vi "HAPS_LoadTable_SetBeam_Manual_Selected.vi"() -> ()   [LabVIEW 2023, in "HAPS.lvlib"]
uses:
  HAPS.lvlib
  set_ele.ctl
  HAPS_SerialPort.ctl
  HAPS_MCU_ELE_Func.ctl
  <vilib>/Utility/file.llb/Read Delimited Spreadsheet (string).vi
  R_S/R_S.lvlib
panel:
  out "error IO":errorcluster
  out "Err_code":i32
  out "status":bool
  in  "offset?":bool
  in  "simu.?":bool
  in  "set_ele":T1={"ch"=0, "chain_id"=0, "group"=0, "array_id"=0, "ele_phase"=0, "ele_gain"=35, "com_gain"=17, "pd_range"=0}
  in  "ele_gain":i32=35
  in  "BFIC_id?":i32
  in  "Group?":i32
  in  "sys reboot?":bool=TRUE
  in  "VISA resource name":refnum<visa-resource-name>="COM1"
  in  "file path":path=path "D:/_Project/_Code/LabVIEW/_CLC_Gen4/CLC_LV2023/CLC_Cali/Log/HAPS/Preset.csv"
  out "Remaining quantity":i32
  out "ele phase":i32
  out "ele gain":i32
  out "channel":i32
  out "chain ID":i32
  out "group":i32
  out "array id":i32
  # "HAPS 24x24 Setting Manual In-Phase : \n                                                           One BFIC"
  # "Tx:35\nRx:22"
  # "Not using!!!!!!!!!!!!!!!!!!!!!!!!!!!!!!!!!!!!!!!!"
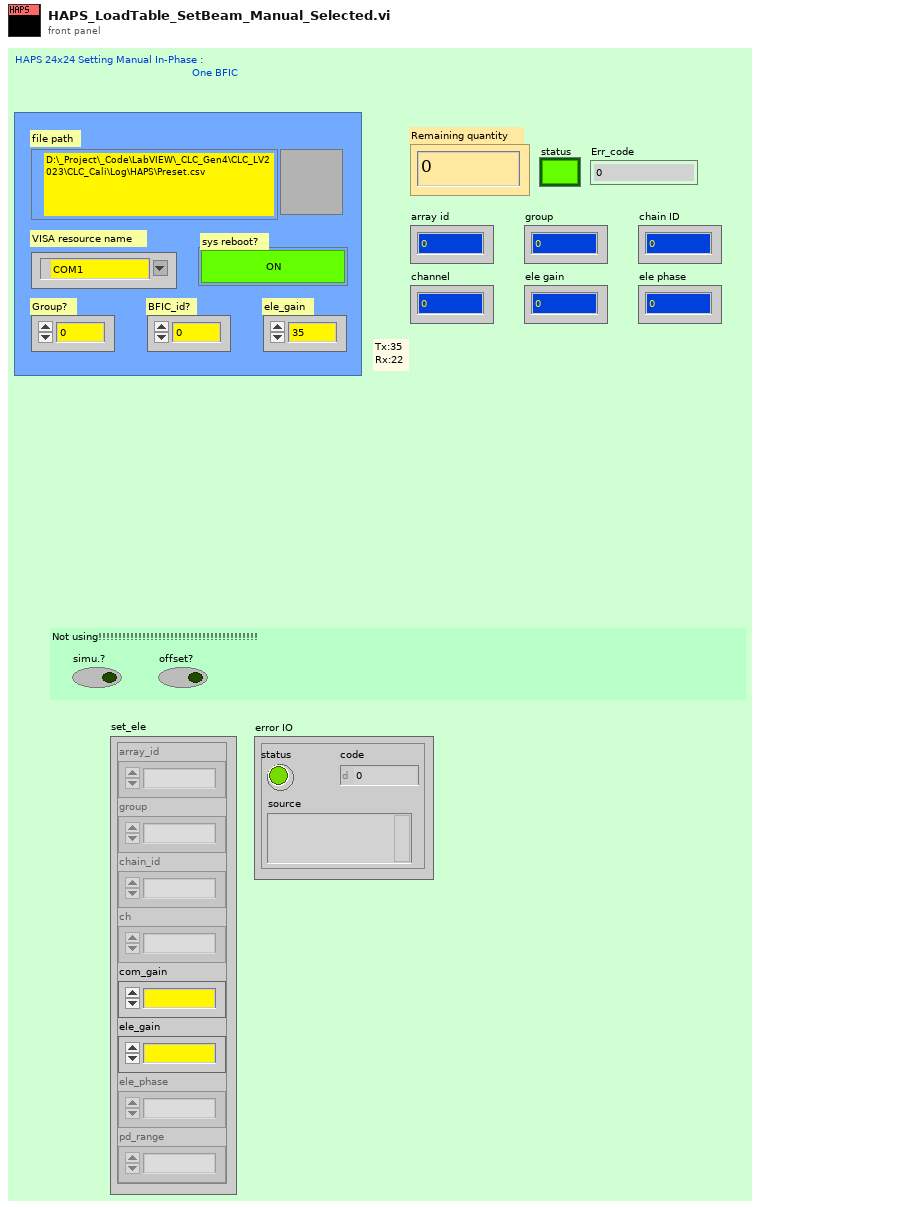
[diagram p1: front panel]
types:
  T1 = typedef "HAPS.lvlib/set_ele.ctl" = cluster{"ch":i32, "chain_id":i32, "group":i32, "array_id":i32, "ele_phase":i32, "ele_gain":i32, "com_gain":i32, "pd_range":i32}
  T2 = typedef "HAPS.lvlib/HAPS_SerialPort.ctl" = enum16{"Init", "Close", "CMD", "Flush"}
  T3 = typedef "HAPS.lvlib/HAPS_MCU_ELE_Func.ctl" = enum16{"array_init", "set_com_gain", "set_ch_gain_phase", "set_pd_range", "get_preamp_temp", "get_bfic_temp", "get_tx_pd", "ch_on", "ch_on_2", "ch_ctrl_all", "array_ctrl_src"}
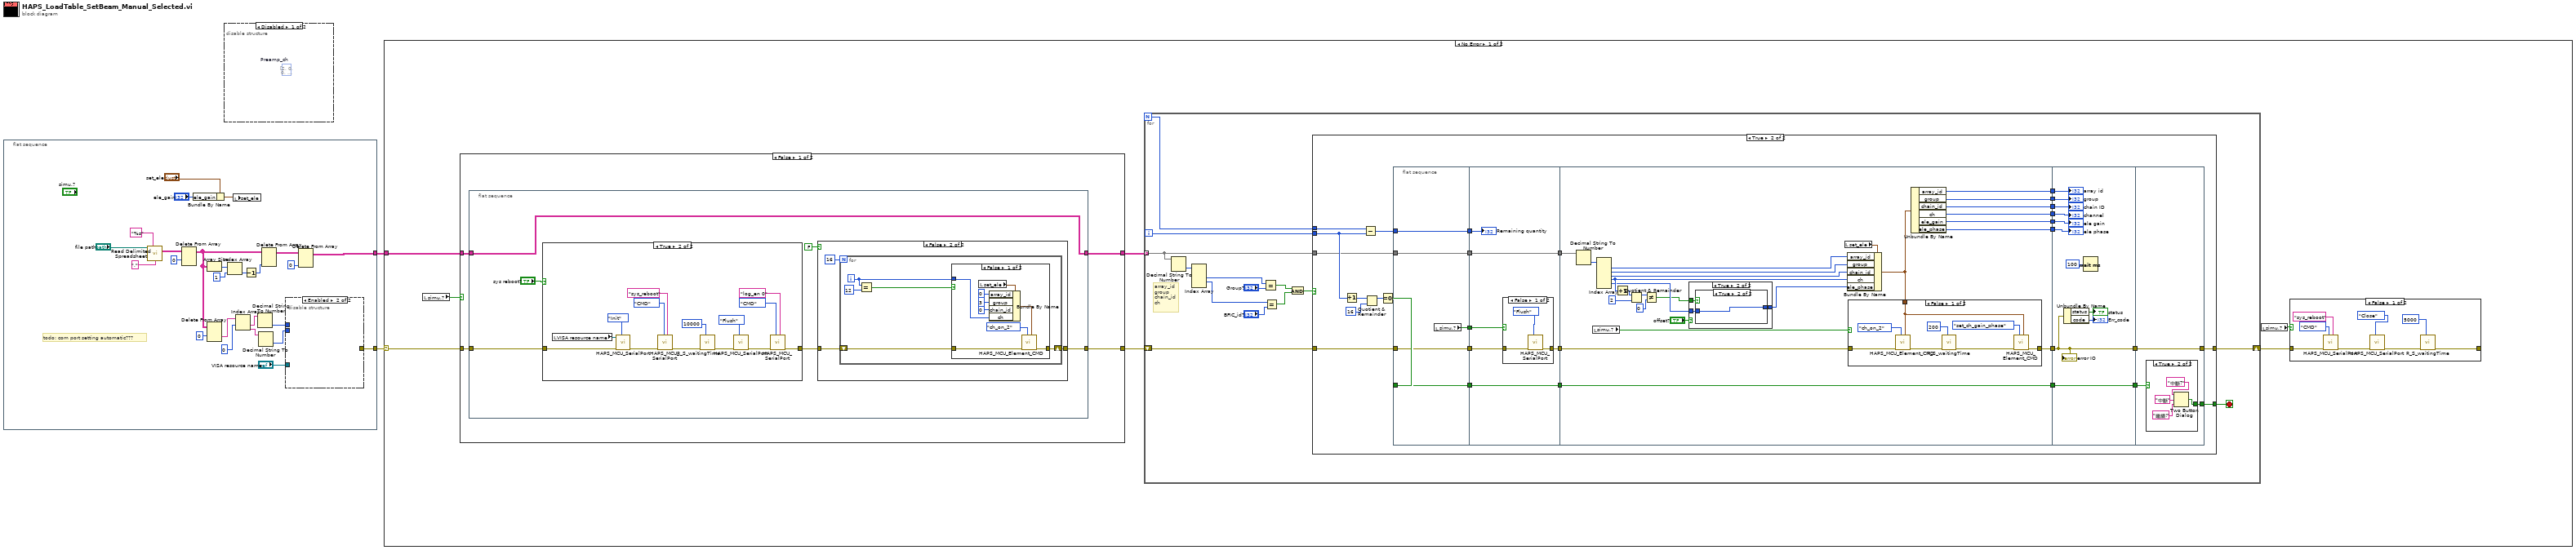
[diagram p0: block diagram]
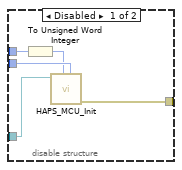
[diagram p2: hidden frame]
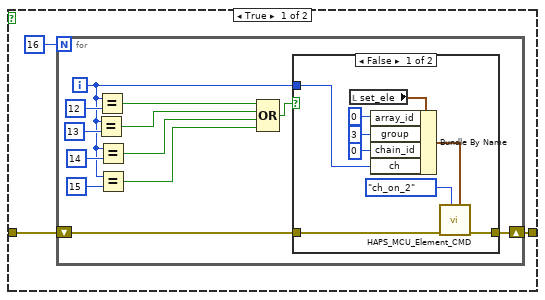
[diagram p5: hidden frame]
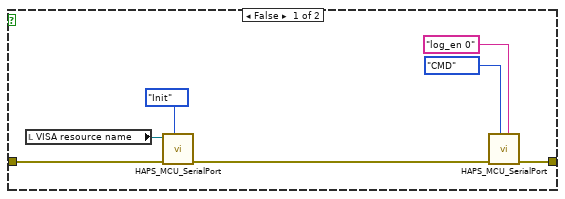
[diagram p8: hidden frame]
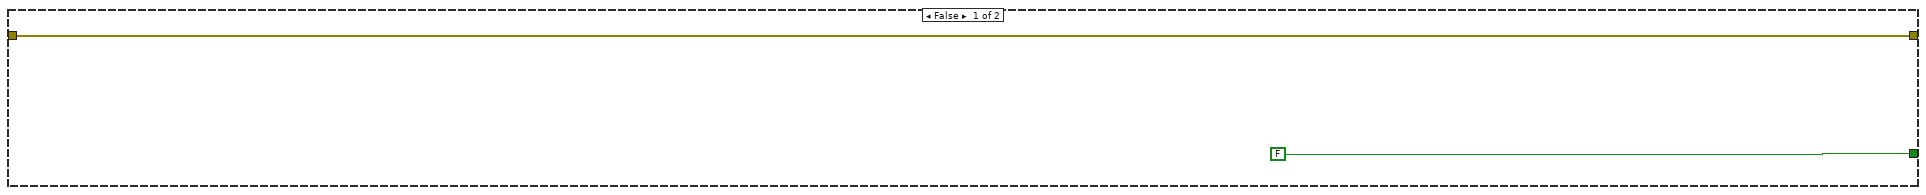
[diagram p10: hidden frame]
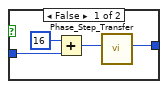
[diagram p13: hidden frame]
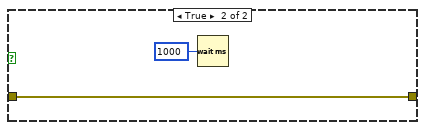
[diagram p14: hidden frame]
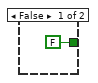
[diagram p15: hidden frame]
diagram:
  n1 = flat-sequence {
    tunnel: [w19] -> w2
    tunnel: [w6] -> w1
    frame #0 {
      # "todo: com port setting automatic???"
      n2 = call-poly <vilib>:"Read Delimited Spreadsheet.vi"("file path (dialog if empty)"="file path", "format (%s)"="%s" ("format (%.3f)"), "delimiter (\\t)"="," ("delimiter (\\t)")) -> ("all rows"=w25:string[][])  [unwired: 7 in, 5 out]
      n3 = Delete From Array(array=w25, index (row)=0) -> (array with subset deleted=w15:string[][])  [unwired: 2 in, 1 out]
      n4 = Bundle By Name(cluster="set_ele", "ele_gain"="ele_gain") -> (w3:T1)
      n5 = Array Size(array=w15) -> (size(s)=w23:i32[])
      n6 = Delete From Array(array=w15, index (row)=0) -> (deleted portion=w14:string[])  [unwired: 2 in, 1 out]
      n7 = Index Array(array=w23, index=1) -> (element=w20:i32)
      n8 = local write "set_ele"(w3) -> ()
      n9 = Index Array(array=w14, index #1=0 ("index")) -> (element #1=w13:string, element #2=w12:string)  [unwired: 1 in]
      n10 = Decrement(x=w20) -> (x-1=w22:i32)
      n11 = Decimal String To Number(string=w13) -> (number=w9:i32)  [unwired: 2 in, 1 out]
      n12 = Decimal String To Number(string=w12) -> (number=w8:i32)  [unwired: 2 in, 1 out]
      n13 = Delete From Array(array=w15, index (col)=w22) -> (array with subset deleted=w18:string[][])  [unwired: 2 in, 1 out]
      n14 = disable-structure shown="Enabled" {
        disable-tunnel: [w32 _] -> w19
        disable-tunnel: w9 -> [w31 _]
        disable-tunnel: w8 -> [w30 _]
        disable-tunnel: "VISA resource name" -> [w29 _]
        frame Disabled {
          n15 = To Unsigned Word Integer(number=w31) -> (unsigned 16bit integer=w28:u16)
          n16 = call "HAPS_MCU_Init.vi"("array_id"=w30, "Tx/Rx"=w28, "VISA resource name"=w29) -> ("error out"=w32:errorcluster)  [unwired: 8 in]
        }
        frame Enabled {
        }
      }
      n17 = Delete From Array(array=w18, index (col)=0 ("index (row)")) -> (array with subset deleted=w6:string[][])  [unwired: 2 in, 1 out]
    }
  }
  n18 = disable-structure shown="Disabled" {
    frame Disabled {
      (unwired) i32[][] [[2, 0, 0, 8, 8, 10, 11, 9, 9, 1, 1, 3], [3, 1, 1, 9, 9, 11, 13, 15, 15, 7, 7, 5], [5, 7, 7, 15, 15, 13, 14, 14, 6, 6, 4, 12]]  # Preamp_ch
    }
    frame Enabled {
    }
  }
  n19 = case shown="No Error" w2 {
    selector: w2 -> [w37 _]
    tunnel: w1 -> [w39 _]
    frame No Error {
      n20 = local read "simu.?"() -> (w35:bool)
      n21 = case shown="False" w35 {
        tunnel: w39 -> [w52 w124]
        tunnel: [w51 w124] -> w38
        tunnel: w37 -> [w50 w123]
        tunnel: [w49 w123] -> w36
        frame False {
          n22 = flat-sequence {
            tunnel: w52 -> [w58]
            tunnel: [w58] -> w51
            tunnel: w50 -> [w56]
            tunnel: [w57] -> w49
            frame #0 {
              n23 = case shown="True" "sys reboot?" {
                tunnel: w56 -> [w106 w120]
                tunnel: [w104 w118] -> w55
                frame False {
                  n24 = local read "VISA resource name"() -> (w102:refnum<visa-resource-name>)
                  n25 = call "HAPS_MCU_SerialPort.vi"("HAPS_SerialPort_Func"=HAPS_SerialPort."Init", "error in"=w106, "VISA resource name"=w102) -> ("error out"=w103:errorcluster)  [unwired: 6 in, 2 out]
                  n26 = call "HAPS_MCU_SerialPort.vi"("Command"="log_en 0", "HAPS_SerialPort_Func"=enum16{"Init", "Close", "CMD"}."CMD" ("HAPS_SerialPort"), "error in"=w103) -> ("error out"=w104:errorcluster)  [unwired: 6 in, 2 out]
                }
                frame True {
                  n27 = local read "VISA resource name"() -> (w109:refnum<visa-resource-name>)
                  n28 = call "HAPS_MCU_SerialPort.vi"("HAPS_SerialPort_Func"=HAPS_SerialPort."Init", "error in"=w120, "VISA resource name"=w109) -> ("error out"=w115:errorcluster)  [unwired: 6 in, 2 out]
                  n29 = call "HAPS_MCU_SerialPort.vi"("Command"="sys_reboot", "HAPS_SerialPort_Func"=enum16{"Init", "Close", "CMD"}."CMD" ("HAPS_SerialPort"), "error in"=w115) -> ("error out"=w114:errorcluster)  [unwired: 6 in, 2 out]
                  n30 = call "R_S_waitingTime.vi"("Waiting Time(ms)"=u32 10000, "error in"=w114) -> ("error out"=w112:errorcluster)  [unwired: 9 in]
                  n31 = call "HAPS_MCU_SerialPort.vi"("HAPS_SerialPort_Func"=HAPS_SerialPort."Flush", "error in"=w112) -> ("error out"=w110:errorcluster)  [unwired: 7 in, 2 out]
                  n32 = call "HAPS_MCU_SerialPort.vi"("Command"="log_en 0", "HAPS_SerialPort_Func"=enum16{"Init", "Close", "CMD"}."CMD" ("HAPS_SerialPort"), "error in"=w110) -> ("error out"=w118:errorcluster)  [unwired: 6 in, 2 out]
                }
              }
              n33 = case shown="False" FALSE {
                tunnel: [w60 w85] -> w57
                tunnel: w55 -> [w59 w84]
                frame True {
                  n34 = for {
                    N: 16 -> [_]
                    shift-right: [w72] -> w60
                    shift-left: w59 -> [w73]
                    i -> [w63]
                    n35 = Equal?(x=w63, y=13) -> (x = y?=w67:bool)
                    n36 = Equal?(x=w63, y=12) -> (x = y?=w71:bool)
                    n37 = Equal?(x=w63, y=14) -> (x = y?=w65:bool)
                    n38 = Equal?(x=w63, y=15) -> (x = y?=w62:bool)
                    n39 = Compound Arithmetic op=OR(w71, w67, w65, w62) -> (w68:bool)
                    n40 = case shown="False" w68 {
                      tunnel: w73 -> [w76 w83]
                      tunnel: [w75 w83] -> w72
                      tunnel: w63 -> [w74 _]
                      frame False {
                        n41 = local read "set_ele"() -> (w78:T1)
                        n42 = Bundle By Name(cluster=w78, "array_id"=0, "group"=3, "chain_id"=0, "ch"=w74) -> (w79:T1)
                        n43 = call "HAPS_MCU_Element_CMD.vi"("set_ele"=w79, "HAPS_MCU_ELE_Func."=HAPS_MCU_ELE_Func."ch_on_2", "error in"=w76) -> ("error out"=w75:errorcluster)  [unwired: 7 in, 1 out]
                      }
                      frame True {
                      }
                    }
                  }
                }
                frame False {
                  n44 = for {
                    N: 16 -> [_]
                    shift-right: [w90] -> w85
                    shift-left: w84 -> [w91]
                    i -> [w88]
                    n45 = Equal?(x=w88, y=12) -> (x = y?=w87:bool)
                    n46 = case shown="False" w87 {
                      tunnel: w91 -> [w94 w101]
                      tunnel: [w93 w101] -> w90
                      tunnel: w88 -> [w92 _]
                      frame False {
                        n47 = local read "set_ele"() -> (w96:T1)
                        n48 = Bundle By Name(cluster=w96, "array_id"=0, "group"=3, "chain_id"=0, "ch"=w92) -> (w97:T1)
                        n49 = call "HAPS_MCU_Element_CMD.vi"("set_ele"=w97, "HAPS_MCU_ELE_Func."=HAPS_MCU_ELE_Func."ch_on_2", "error in"=w94) -> ("error out"=w93:errorcluster)  [unwired: 7 in, 1 out]
                      }
                      frame True {
                      }
                    }
                  }
                }
              }
            }
          }
        }
        frame True {
        }
      }
      n50 = for {
        N -> [w136]
        tunnel: w38 -> [w133] mode=indexing
        shift-right: [w138] -> w33
        shift-left: w36 -> [w137]
        i -> [w135]
        stop <- w132 stop-if-true
        # "array_id\ngroup\nchain_id\nch"
        n51 = Decimal String To Number(string=w133) -> (number=w134:i32[])  [unwired: 2 in, 1 out]
        n52 = Index Array(array=w134) -> (element #2=w131:i32, element #3=w129:i32)  [unwired: 4 in, 2 out]
        n53 = Equal?(x=w131, y="Group?") -> (x = y?=w127:bool)
        n54 = Equal?(x=w129, y="BFIC_id?") -> (x = y?=w126:bool)
        n55 = Compound Arithmetic op=AND(w127, w126) -> (w125:bool)
        n56 = case shown="True" w125 {
          tunnel: [w139 w152] -> w138
          tunnel: w137 -> [w139 w151]
          tunnel: w136 -> [_ w150]
          tunnel: w135 -> [_ w149]
          tunnel: w133 -> [_ w148]
          tunnel: [FALSE ("T button?") w142] -> w132
          frame False {
          }
          frame True {
            n57 = Increment(x=w149) -> (x+1=w146:i32)
            n58 = Subtract(x=w150, y=w149) -> (x-y=w147:i32)
            n59 = Quotient & Remainder(x=w146, y=16) -> (x-y*floor(x/y)=w144:i32)  [unwired: 1 out]
            n60 = Equal To 0?(x=w144) -> (x = 0?=w143:bool)
            n61 = flat-sequence {
              tunnel: w147 -> [w172]
              tunnel: w151 -> [w173]
              tunnel: w148 -> [w174]
              tunnel: [w174] -> w169
              tunnel: [w173] -> w168
              tunnel: [w172] -> w167
              tunnel: w143 -> [w171]
              tunnel: [w171] -> w166
              tunnel: [w170] -> w141
              tunnel: [w179] -> w165
              tunnel: [w178] -> w164
              tunnel: w169 -> [w179]
              tunnel: w168 -> [w177]
              tunnel: w167 -> [w180]
              tunnel: w166 -> [w176]
              tunnel: [w176] -> w163
              tunnel: w141 -> [w175]
              tunnel: w165 -> [w210]
              tunnel: w164 -> [w208]
              tunnel: [w196] -> w162
              tunnel: [w206] -> w161
              tunnel: [w205] -> w160
              tunnel: [w204] -> w159
              tunnel: [w203] -> w158
              tunnel: [w202] -> w157
              tunnel: [w201] -> w156
              tunnel: w163 -> [w197]
              tunnel: [w197] -> w155
              tunnel: w162 -> [w232]
              tunnel: w161 -> [w240]
              tunnel: w160 -> [w239]
              tunnel: w159 -> [w238]
              tunnel: w158 -> [w237]
              tunnel: w157 -> [w236]
              tunnel: w156 -> [w235]
              tunnel: [w232] -> w154
              tunnel: w155 -> [w233]
              tunnel: [w233] -> w153
              tunnel: w154 -> [w243]
              tunnel: w153 -> [w242]
              tunnel: [w243] -> w152
              tunnel: [w241] -> w142
              frame #0 {
                n62 = local read "simu.?"() -> (w170:bool)
              }
              frame #1 {
                n63 = case shown="False" w175 {
                  tunnel: [w183 w184] -> w178
                  tunnel: w177 -> [w182 w184]
                  frame False {
                    n64 = call "HAPS_MCU_SerialPort.vi"("HAPS_SerialPort_Func"=HAPS_SerialPort."Flush", "error in"=w182) -> ("error out"=w183:errorcluster)  [unwired: 7 in, 2 out]
                  }
                  frame True {
                  }
                }
                "Remaining quantity" <- w180
              }
              frame #2 {
                n65 = Decimal String To Number(string=w210) -> (number=w209:i32[])  [unwired: 2 in, 1 out]
                n66 = local read "simu.?"() -> (w195:bool)
                n67 = Index Array(array=w209) -> (element #1=w207:i32, element #2=w200:i32, element #3=w199:i32, element #4=w193:i32, element #5=w189:i32)  [unwired: 6 in, 1 out]
                n68 = Increment(x=w193) -> (x+1=w185:i32)
                n69 = Quotient & Remainder(x=w185, y=2) -> (x-y*floor(x/y)=w191:i32)  [unwired: 1 out]
                n70 = Not Equal?(x=w191, y=0) -> (x != y?=w188:bool)
                n71 = case shown="True" "offset?" {
                  tunnel: w189 -> [w211 w214]
                  tunnel: w188 -> [_ w213]
                  tunnel: [w211 w212] -> w187
                  frame False {
                  }
                  frame True {
                    n72 = case shown="True" w213 {
                      tunnel: w214 -> [w218 w219]
                      tunnel: [w215 w219] -> w212
                      frame False {
                        n73 = Add(x=16, y=w218) -> (x+y=w216:i32)
                        n74 = call "Phase_Step_Transfer.vi"("Input_Phase_Step"=w216) -> ("Output_Phase_Step"=w215:i32)  [unwired: 10 in]
                      }
                      frame True {
                      }
                    }
                  }
                }
                n75 = local read "set_ele"() -> (w198:T1)
                n76 = Bundle By Name(cluster=w198, "array_id"=w207, "group"=w200, "chain_id"=w199, "ch"=w193, "ele_phase"=w187) -> (w194:T1)
                n77 = case shown="False" w195 {
                  tunnel: w208 -> [w227 w229]
                  tunnel: w194 -> [w226 _]
                  tunnel: [w225 w229] -> w196
                  frame False {
                    n78 = call "HAPS_MCU_Element_CMD.vi"("set_ele"=w226, "HAPS_MCU_ELE_Func."=HAPS_MCU_ELE_Func."ch_on_2", "error in"=w227) -> ("error out"=w221:errorcluster)  [unwired: 7 in, 1 out]
                    n79 = call "R_S_waitingTime.vi"("Waiting Time(ms)"=u32 200, "error in"=w221) -> ("error out"=w220:errorcluster)  [unwired: 9 in]
                    n80 = call "HAPS_MCU_Element_CMD.vi"("set_ele"=w226, "HAPS_MCU_ELE_Func."=HAPS_MCU_ELE_Func."set_ch_gain_phase", "error in"=w220) -> ("error out"=w225:errorcluster)  [unwired: 7 in, 1 out]
                  }
                  frame True {
                    n81 = Wait (ms)(milliseconds to wait=u32 1000) -> ()  [unwired: 1 out]
                  }
                }
                n82 = Unbundle By Name(w194) -> ("array_id"=w206:i32, "group"=w205:i32, "chain_id"=w204:i32, "ch"=w203:i32, "ele_gain"=w202:i32, "ele_phase"=w201:i32)
              }
              frame #3 {
                n83 = Unbundle By Name(w232) -> ("status"=→"status":bool, "code"=→"Err_code":i32)
                n84 = Wait (ms)(milliseconds to wait=u32 100) -> ()  [unwired: 1 out]
                "group" <- w239
                "chain ID" <- w238
                "channel" <- w237
                "ele gain" <- w236
                "ele phase" <- w235
                "array id" <- w240
                "error IO" <- w232
              }
              frame #4 {
                n85 = case shown="True" w242 {
                  tunnel: [FALSE ("T button?") w245] -> w241
                  frame False {
                  }
                  frame True {
                    n86 = Two Button Dialog(message="中斷?", 1:"繼續!" ("F button name (\"Cancel\")"), 2:"中斷" ("T button name (\"OK\")")) -> (T button?=w245:bool)
                  }
                }
              }
            }
          }
        }
      }
      n87 = local read "simu.?"() -> (w34:bool)
      n88 = case shown="False" w34 {
        tunnel: [w40 w48] -> _
        tunnel: w33 -> [w47 w48]
        frame False {
          n89 = call "HAPS_MCU_SerialPort.vi"("Command"="sys_reboot", "HAPS_SerialPort_Func"=enum16{"Init", "Close", "CMD"}."CMD" ("HAPS_SerialPort"), "error in"=w47) -> ("error out"=w43:errorcluster)  [unwired: 6 in, 2 out]
          n90 = call "HAPS_MCU_SerialPort.vi"("HAPS_SerialPort_Func"=HAPS_SerialPort."Close", "error in"=w43) -> ("error out"=w41:errorcluster)  [unwired: 7 in, 2 out]
          n91 = call "R_S_waitingTime.vi"("Waiting Time(ms)"=u32 5000, "error in"=w41) -> ("error out"=w40:errorcluster)  [unwired: 9 in]
        }
        frame True {
        }
      }
    }
    frame Error {
    }
  }
